vi "Waypoint_Packet_Creator.vi"(1 "Request Type":enum16{"Append to End", "Replace List"}(ring), 2 "Waypoint List":T1(array[cluster]) {"Longitude" format="%#_15g"; "Latitude" format="%#_15g"}) -> (0 "Waypoint Packet":string)   [LabVIEW 2009]
panel:
  out "# of WPTS":u8
  out "alt":u16
  out "checksum string":string
  out "Checksum":u32
  out "Waypoint Packet HEX":string
  out "alt string":string
  out "longitude string":string
  out "latitude string":string
  out "lon":i32
  out "lat":i32
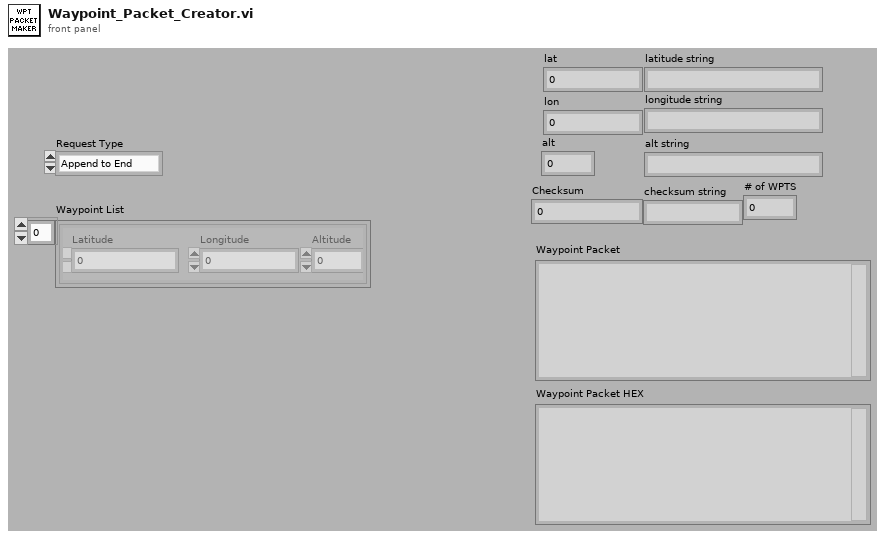
[diagram p1: front panel]
types:
  T1 = cluster{"Latitude":dbl, "Longitude":dbl, "Altitude":u16}[]
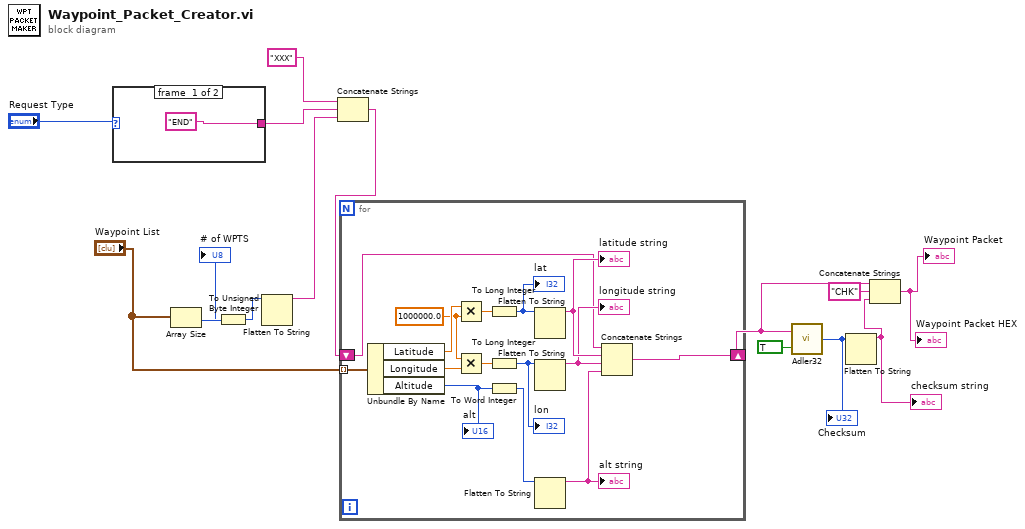
[diagram p0: block diagram]
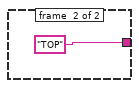
[diagram p2: hidden frame]
diagram:
  n1 = case shown="\"Append to End\", Default" "Request Type" {
    tunnel: ["END" "TOP"] -> w12
    frame #0 {
    }
    frame #1 {
    }
  }
  n2 = Array Size(array="Waypoint List") -> (size(s)=w3:i32)
  n3 = To Unsigned Byte Integer(number=w3) -> (unsigned 8bit integer=w2:u8)
  "# of WPTS" <- w2
  n4 = Flatten To String(anything=w2) -> (data string=w1:string)  [unwired: 3 in, 2 out]
  n5 = Concatenate Strings("XXX", w12, w1) -> (w11:string)
  n6 = for {
    tunnel: "Waypoint List" -> [w31] mode=indexing
    shift-right: [w20] -> w8
    shift-left: w11 -> [w17]
    w29 = 1000000.0 ("y")
    n7 = Unbundle By Name(w31) -> ("Latitude"=w30:dbl, "Longitude"=w28:dbl, "Altitude"=w19:u16)
    "alt" <- w19
    n8 = Multiply(x=w30, y=w29) -> (x*y=w27:dbl)
    n9 = Multiply(x=w29, y=w28) -> (x*y=w26:dbl)
    n10 = To Long Integer(number=w27) -> (32bit integer=w25:i32)
    "lat" <- w25
    n11 = To Long Integer(number=w26) -> (32bit integer=w24:i32)
    "lon" <- w24
    n12 = To Word Integer(number=w19) -> (16bit integer=w18:i16)
    n13 = Flatten To String(anything=w25) -> (data string=w23:string)  [unwired: 3 in, 2 out]
    "latitude string" <- w23
    n14 = Flatten To String(anything=w24) -> (data string=w22:string)  [unwired: 3 in, 2 out]
    "longitude string" <- w22
    n15 = Flatten To String(anything=w18) -> (data string=w21:string)  [unwired: 3 in, 2 out]
    "alt string" <- w21
    n16 = Concatenate Strings(w17, w23, w22, w21) -> (w20:string)
  }
  n17 = call "Adler32.vi"("Modulus?"=TRUE, "String"=w8) -> ("Checksum"=w10:u32)
  "Checksum" <- w10
  n18 = Flatten To String(anything=w10) -> (data string=w6:string)  [unwired: 3 in, 2 out]
  "checksum string" <- w6
  n19 = Concatenate Strings(w8, "CHK" ("string"), w6) -> (→"Waypoint Packet" →"Waypoint Packet HEX":string)
